vi "Set cif_pluginloader_DiscoveredPlugins.vi"(7 "Complete Call (T)":bool=TRUE, 8 "error in (no error)":errorcluster, 10 "package_templatemessage":T1, 11 "gRPCid":T6) -> (0 "error out":errorcluster)   [LabVIEW 2021, in "CIF_PluginLoader_server.lvlib"]
uses:
  CIF_PluginLoader_server.lvlib
  <vilib>/gRPC/LabVIEW gRPC Library/Shared/grpcId.ctl
  cif_pluginloader_DiscoveredPlugins.ctl
  cif_pluginloader_DiscoveredPlugin.ctl
  cif_common_Version.ctl
  cif_manager_PluginMetadata.ctl
  cif_common_Status.ctl
  cif_pluginloader_DiscoveredPlugins_Flat.ctl
  cif_pluginloader_DiscoveredPlugin_Flat.ctl
  cif_common_Version_Flat.ctl
  cif_manager_PluginMetadata_Flat.ctl
  cif_common_Status_Flat.ctl
  dcc74a39-081a-4bdd-860b-8ed792803c96.vi
  RichToFlatcif_pluginloader_DiscoveredPlugin.vi
  RichToFlatcif_common_Status.vi
  <vilib>/gRPC/LabVIEW gRPC Library/Shared/TranslateGrpcError.vi
  RichToFlatcif_common_Version.vi
  RichToFlatcif_manager_PluginMetadata.vi
  <vilib>/gRPC/LabVIEW gRPC Library/Server API/Server/Get Server DLL Path.vi
  <vilib>/Utility/error.llb/Error Cluster From Error Code.vi
  <vilib>/gRPC/LabVIEW gRPC Library/grpc-lvsupport-release.lvlib
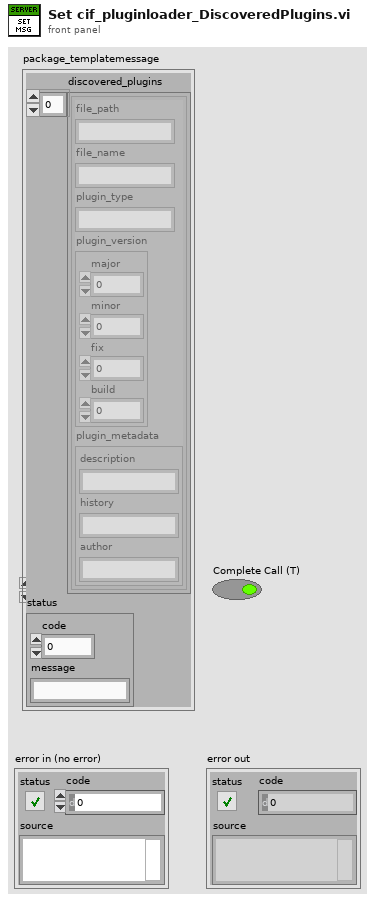
[diagram p1: front panel]
types:
  T1 = typedef "CIF_PluginLoader_server.lvlib/cif_pluginloader_DiscoveredPlugins.ctl" = cluster{"discovered_plugins":T2[], "status":T5}
  T2 = typedef "CIF_PluginLoader_server.lvlib/cif_pluginloader_DiscoveredPlugin.ctl" = cluster{"file_path":string, "file_name":string, "plugin_type":string, "plugin_version":T3, "plugin_metadata":T4}
  T3 = typedef "CIF_PluginLoader_server.lvlib/cif_common_Version.ctl" = cluster{"major":u32, "minor":u32, "fix":u32, "build":u32}
  T4 = typedef "CIF_PluginLoader_server.lvlib/cif_manager_PluginMetadata.ctl" = cluster{"description":string, "history":string, "author":string}
  T5 = typedef "CIF_PluginLoader_server.lvlib/cif_common_Status.ctl" = cluster{"code":i32, "message":string}
  T6 = typedef "grpc-lvsupport-release.lvlib/grpcId.ctl" = u64
  T7 = typedef "CIF_PluginLoader_server.lvlib/cif_pluginloader_DiscoveredPlugins_Flat.ctl" = cluster{"discovered_plugins":T8[], "status":T11}
  T8 = typedef "CIF_PluginLoader_server.lvlib/cif_pluginloader_DiscoveredPlugin_Flat.ctl" = cluster{"file_path":string, "file_name":string, "plugin_type":string, "plugin_version":T9, "plugin_metadata":T10}
  T9 = typedef "CIF_PluginLoader_server.lvlib/cif_common_Version_Flat.ctl" = cluster{"major":u32, "minor":u32, "fix":u32, "build":u32}
  T10 = typedef "CIF_PluginLoader_server.lvlib/cif_manager_PluginMetadata_Flat.ctl" = cluster{"description":string, "history":string, "author":string}
  T11 = typedef "CIF_PluginLoader_server.lvlib/cif_common_Status_Flat.ctl" = cluster{"code":i32, "message":string}
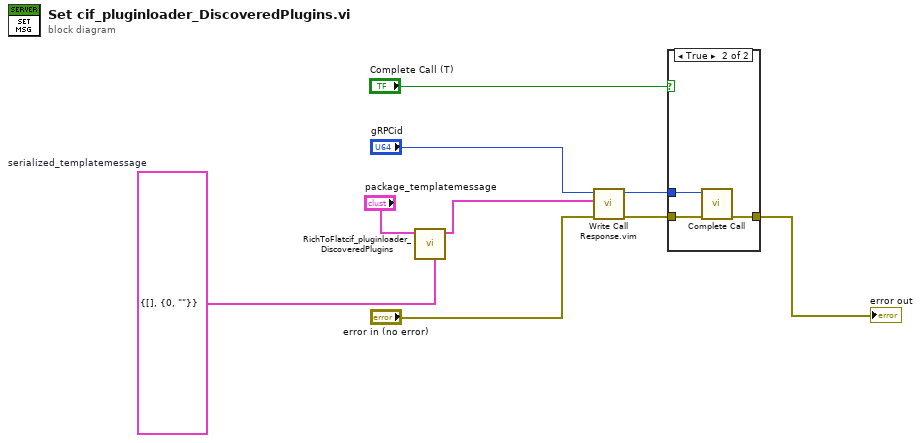
[diagram p0: block diagram]
diagram:
  w2 = T7 {"discovered_plugins"=[], "status"={"code"=0, "message"=""}}  # serialized_templatemessage
  n1 = call "RichToFlatcif_pluginloader_DiscoveredPlugins.vi"("OutputClusterType"=w2, "InputCluster"="package_templatemessage") -> ("OutputCluster"=w1:T7)  [unwired: 9 in]
  n2 = call "Write Call Response.vim"("error in"="error in (no error)", "Response Data"=w1, "gRPCid in"="gRPCid") -> ("error out"=w6:errorcluster, "gRPCid out"=w7:T6)  [unwired: 7 in]
  n3 = case shown="True" "Complete Call (T)" {
    tunnel: [w10 w13] -> w9
    tunnel: w7 -> [_ w12]
    tunnel: w6 -> [w10 w11]
    frame False {
    }
    frame True {
      n4 = call <vilib>:"Complete Call.vi"("gRPCid"=w12, "error in"=w11) -> ("error out"=w13:errorcluster)  [unwired: 8 in]
    }
  }
  "error out" <- w9
